vi "Get Endpoint.vi"(8 "error in (no error)":errorcluster, 11 "WebSocket Connection in":refnum<class "WebSocket Connection.lvclass">) -> (0 "error out":errorcluster, 1 "remote port":u16, 2 "remote address":string, 3 "WebSocket Connection out":refnum<class "WebSocket Connection.lvclass">)   [LabVIEW 2019, in "WebSocket Server Toolkit.lvlib" / "WebSocket Connection.lvclass"]
doc: "<b>Description</b> Gets the remote endpoint of the current connection.\n\n<b>Outputs</b>\n<b>remote address</b>: The address associated with the remote endpoint.\n<b>remote port</b>: The port associated with the remote endpoint."
uses:
  WebSocket Connection.lvclass
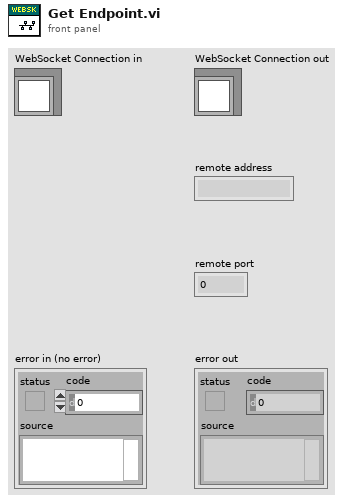
[diagram p1: front panel]
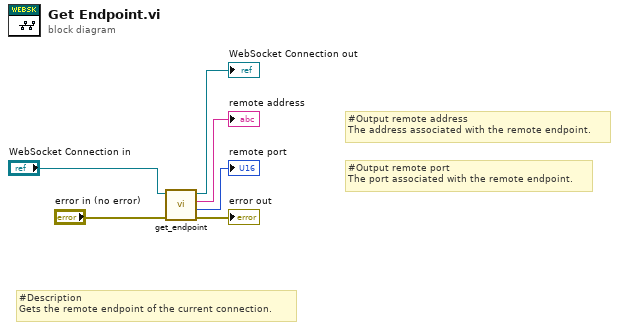
[diagram p0: block diagram]
diagram:
  # "#Output remote address\nThe address associated with the remote endpoint."
  # "#Output remote port\nThe port associated with the remote endpoint."
  # "#Description\nGets the remote endpoint of the current connection."
  n1 = call-dynamic "get_endpoint.vi"("error in (no error)"="error in (no error)", "WebSocket Connection in"="WebSocket Connection in") -> ("error out"=→"error out":errorcluster, "remote port"=→"remote port":u16, "remote address"=→"remote address":string, "WebSocket Connection out"=→"WebSocket Connection out":refnum<class "WebSocket Connection.lvclass">)  [unwired: 6 in]
